vi "USB Scan Device.vi"(11 "pDevHandle":i32) -> (2 "function return":i32, 3 "pDevHandle out":i32)   [LabVIEW 2010, in "usb_device.lvlib"]
doc: "int WINAPI USB_ScanDevice(int *pDevHandle,int *pFd,int DevNum);"
uses:
  usb_device.lvlib
  USB2XXX/trunk/USB2XXX/USB2XXX/vs2010/Release/USB2XXX.dll
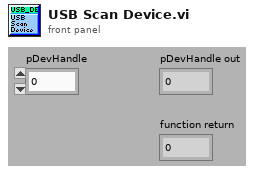
[diagram p1: front panel]
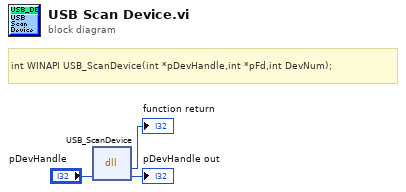
[diagram p0: block diagram]
diagram:
  # "int WINAPI USB_ScanDevice(int *pDevHandle,int *pFd,int DevNum);"
  n1 = dll-call lib="E:/Projects/USB2XXX/trunk/USB2XXX/USB2XXX/vs2010/Release/USB2XXX.*" fn="USB_ScanDevice"("pDevHandle"="pDevHandle") -> (→"function return":i32, "pDevHandle"=→"pDevHandle out":i32)  [unwired: 3 in, 2 out]
